vi "Reset old test Values (SubVI).vi"(8 "error in":errorcluster, 9 "Atr in":refnum<vi>, 11 "Test Paragraph":string) -> (0 "error out":errorcluster)   [LabVIEW 2017]
uses:
  <vilib>/Utility/miscctls.llb/LVRowAndColumnTypeDef.ctl
panel:
  out "concatenated string":string
  out "Value":string[][](array[string])
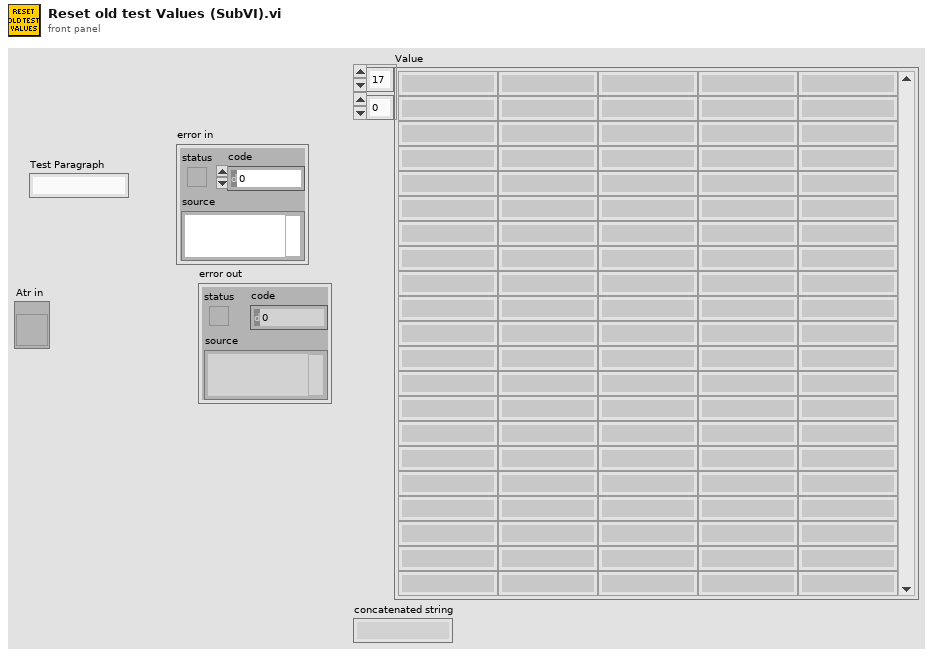
[diagram p1: front panel]
types:
  T1 = typedef "LVRowAndColumnTypeDef.ctl" = cluster{"Row":i32, "Column":i32}
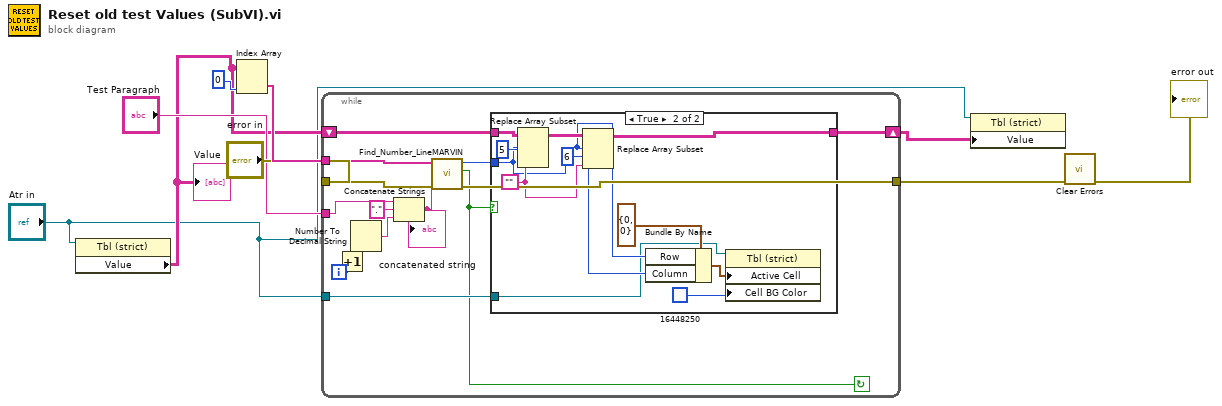
[diagram p0: block diagram]
diagram:
  n1 = property class="Tbl (strict)"(reference="Atr in") -> ("Value"=w4:string[][])  [unwired: 1 in, 2 out]
  "Value" <- w4
  n2 = Index Array(array=w4, index (col)=0 ("disabled index (col)")) -> (element=w8:string[])  [unwired: 1 in]
  n3 = while {
    tunnel: w8 -> [w23]
    tunnel: "Test Paragraph" -> [w20]
    tunnel: "error in" -> [w22]
    tunnel: [w21] -> w6
    shift-right: [w16] -> w2
    shift-left: w4 -> [w15]
    tunnel: "Atr in" -> [w12]
    i -> [w14]
    stop <- w11 continue-if-true
    n4 = Increment(x=w14) -> (x+1=w10:i32)
    n5 = Number To Decimal String(number=w10) -> (decimal integer string=w18:string)  [unwired: 1 in]
    n6 = Concatenate Strings(w20, "." ("string"), w18) -> (w17:string)
    "concatenated string" <- w17
    n7 = call "Find_Number_LineMARVIN.vi"("Test Paragraph"=w17, "error in"=w22, "Row Headers[]"=w23) -> ("error out"=w21:errorcluster, "Found"=w11:bool, "Line number"=w13:i32)  [unwired: 2 in, 1 out]
    n8 = case shown="True" w11 {
      tunnel: [w24 w34] -> w16
      tunnel: w15 -> [w24 w33]
      tunnel: w13 -> [_ w28]
      tunnel: w12 -> [_ w25]
      frame False {
      }
      frame True {
        w31 = ""
        w27 = 6 ("disabled index (col)")
        n9 = Replace Array Subset(array=w33, new element=w31, index (row)=w28, index (col)=5 ("disabled index (col)")) -> (w35:string[][])
        n10 = Replace Array Subset(array=w35, new element=w31, index (row)=w28, index (col)=w27) -> (w34:string[][])
        n11 = Bundle By Name(cluster=T1 {"Row"=0, "Column"=0} ("Active Cell:Active Cell"), "Row"=w28, "Column"=w27) -> (w30:T1)
        n12 = property class="Tbl (strict)"(reference=w25, "Active Cell"=w30, "Cell BG Color"=u32 16448250) -> ()  [unwired: 1 in, 2 out]
      }
    }
  }
  n13 = property class="Tbl (strict)"(reference="Atr in", "Value"=w2) -> ()  [unwired: 1 in, 2 out]
  n14 = call <vilib>:"Clear Errors.vi"("error in (no error)"=w6) -> ("error out"=→"error out":errorcluster)  [unwired: 5 in, 1 out]
